vi "Stepper_test_1.vi"() -> ()   [LabVIEW 2016]
uses:
  <vilib>/myRIO/Instrument Drivers/Onboard IO/DIO/typedefs/DIO Reference.ctl
  <vilib>/myRIO/Common/Instrument Driver Framework/Utilities/typedefs/myRIO Generic Hardware Reference.ctl
  <vilib>/myRIO/Common/Instrument Driver Framework/Utilities/typedefs/Hardware Version Enum.ctl
  <vilib>/myRIO/Common/Instrument Driver Framework/Utilities/typedefs/myRIO v1.0 Reference.ctl
  <vilib>/myRIO/Common/Instrument Driver Framework/Utilities/typedefs/Generic FPGA Reference.ctl
  <vilib>/myRIO/Common/Instrument Driver Framework/myRIO v1.0/DIO/typedefs/DIO Channels List.ctl
  <vilib>/myRIO/Common/Instrument Driver Framework/myRIO v1.0/DIO/typedefs/DIO Channels Enum.ctl
  <vilib>/userdefined/High Color/nirio_resource_hc.ctl
  <vilib>/myRIO/Instrument Drivers/Onboard IO/AI/typedefs/AI Reference.ctl
  <vilib>/myRIO/Common/Instrument Driver Framework/myRIO v1.0/AI/typedefs/AI Channels List.ctl
  <vilib>/myRIO/Common/Instrument Driver Framework/myRIO v1.0/AI/typedefs/AI Channels Enum.ctl
  <vilib>/myRIO/Common/Instrument Driver Framework/Utilities/typedefs/Analog Scaling Constants List.ctl
  <vilib>/myRIO/Common/Instrument Driver Framework/Utilities/typedefs/Analog Scaling Constants.ctl
  <vilib>/myRIO/Common/Instrument Driver Framework/Utilities/vis/Is FPGA Ref Available.vi
  <vilib>/myRIO/Common/Instrument Driver Framework/myRIO v1.0/AI/vis/myRIO v1.1 Open AI.vi
  <vilib>/myRIO/Instrument Drivers/Onboard IO/AI/vis/Read.vi
  <vilib>/myRIO/Common/Instrument Driver Framework/myRIO v1.0/DIO/vis/myRIO v1.1 Open DIO.vi
  <vilib>/myRIO/Instrument Drivers/Onboard IO/DIO/vis/Write.vi
  <vilib>/myRIO/Common/Instrument Driver Framework/Utilities/vis/Validate Channels.vi
  <vilib>/myRIO/Common/Instrument Driver Framework/myRIO v1.0/AI/vis/myRIO v1.0 Reserve AI.vi
  <vilib>/myRIO/Common/Instrument Driver Framework/myRIO v1.0/DIO/vis/myRIO v1.0 Reserve DIO.vi
  <vilib>/myRIO/Common/Instrument Driver Framework/myRIO v1.0/PWM/vis/myRIO v1.1 Open PWM.vi
  <vilib>/myRIO/Common/Instrument Driver Framework/myRIO v1.0/AI/vis/myRIO v1.0 Build MUX Configuration AI.vi
  <vilib>/myRIO/Common/Instrument Driver Framework/myRIO v1.0/Resource Manager/vis/myRIO v1.0 Reserve Channel List.vi
  <vilib>/myRIO/Common/Instrument Driver Framework/myRIO v1.0/DIO/vis/myRIO v1.0 Build MUX Configuration DIO.vi
  <vilib>/myRIO/Common/Instrument Driver Framework/myRIO v1.0/PWM/vis/myRIO v1.0 Reserve PWM.vi
  <vilib>/myRIO/Common/Instrument Driver Framework/myRIO v1.0/Resource Manager/vis/myRIO v1.0 Reserve Channel.vi
  <vilib>/myRIO/Common/Instrument Driver Framework/myRIO v1.0/Resource Manager/vis/myRIO v1.0 Unreserve Channel.vi
  <vilib>/myRIO/Common/Instrument Driver Framework/myRIO v1.0/Resource Manager/vis/myRIO v1.0 Create Configuration List.vi
  <vilib>/myRIO/Common/Instrument Driver Framework/myRIO v1.0/PWM/vis/myRIO v1.0 Build MUX Configuration PWM.vi
  <vilib>/myRIO/Common/Instrument Driver Framework/myRIO v1.0/Resource Manager/vis/myRIO v1.0 Build Mutex Name.vi
  <vilib>/Utility/VariantDataType/GetNumericInfo.vi
  <vilib>/Utility/error.llb/Error Cluster From Error Code.vi
  <vilib>/myRIO/Common/Instrument Driver Framework/myRIO v1.0/myRIO v1.1 Open.vi
  <vilib>/myRIO/Common/Instrument Driver Framework/Utilities/vis/IO Manager.vi
  <vilib>/myRIO/Common/Instrument Driver Framework/Utilities/vis/Configuration Manager.vi
  <vilib>/myRIO/Common/Instrument Driver Framework/myRIO v1.0/Resource Manager/vis/myRIO v1.0 Configure IO.vi
  <vilib>/myRIO/Common/Instrument Driver Framework/myRIO v1.0/myRIO v1.0 Close.vi
  <vilib>/myRIO/Common/Instrument Driver Framework/myRIO v1.0/DIO/vis/myRIO v1.0 Write DIO.vi
  <vilib>/myRIO/Common/Instrument Driver Framework/myRIO v1.0/PWM/vis/myRIO v1.0 Write PWM.vi
  <vilib>/myRIO/Common/Instrument Driver Framework/myRIO v1.0/AI/vis/myRIO v1.0 Get Scaling Constants AI.vi
  <vilib>/myRIO/Common/Instrument Driver Framework/myRIO v1.0/AI/vis/myRIO v1.0 Read AI.vi
  <vilib>/myRIO/Express VI/Onboard IO/DO/DO Express VI.xnode
  <vilib>/myRIO/Instrument Drivers/Onboard IO/DIO/vis/myRIO DIO Open.xnode
  <vilib>/myRIO/Express VI/Onboard IO/AI/AI Express VI.xnode
  <vilib>/myRIO/Instrument Drivers/Onboard IO/AI/vis/myRIO AI Open.xnode
  <vilib>/myRIO/Instrument Drivers/Onboard IO/AI/AI.lvlib
  <vilib>/myRIO/Instrument Drivers/Onboard IO/DIO/DIO.lvlib
  <vilib>/myRIO/Instrument Drivers/Onboard IO/PWM/PWM.lvlib
panel:
  in  "Servo":bool
  in  "PWM channel":tag="B/PWM0"
  out "position [%FS]":dbl(slide) scale=0.0..180.0 scale format="%#_5g"
  out "pulse width [ms]":dbl=1.5
  out "duty cycle [%]":dbl
  out "FSR VALUE":dbl
  in  "RUN":bool
  in  "CLOSE":bool
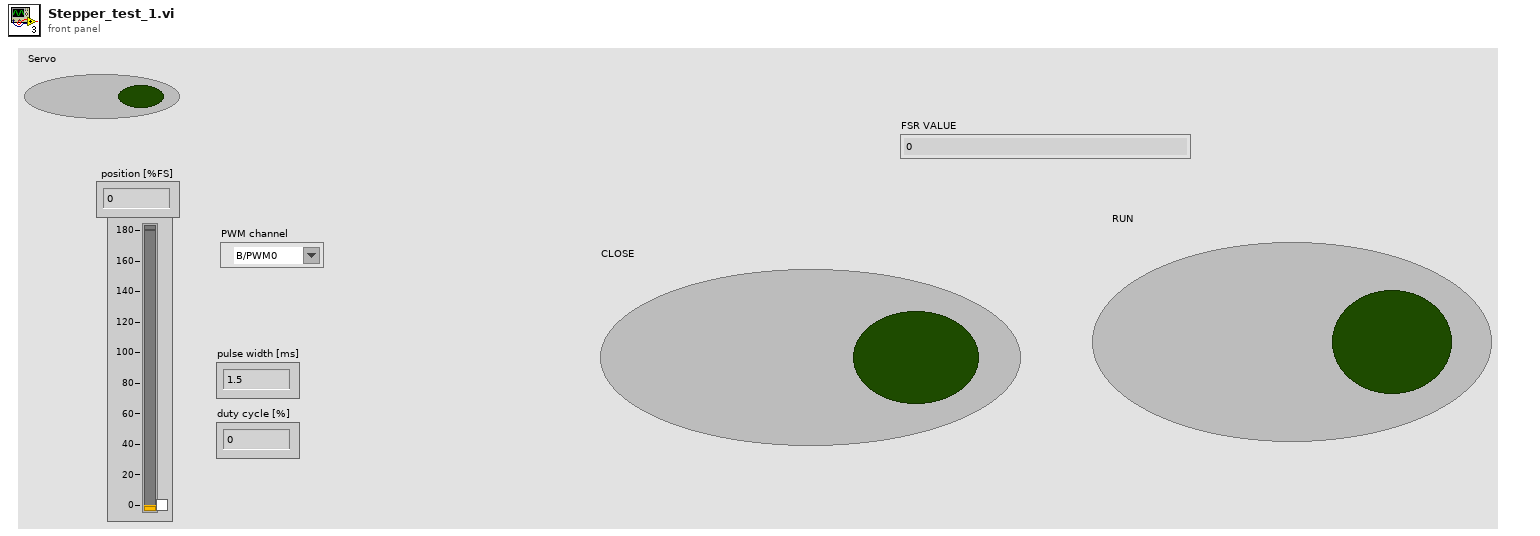
[diagram p1: front panel]
types:
  T1 = typedef "DIO.lvlib/DIO Reference.ctl" = cluster{"myRIO Reference":T2, "DIO Channels List":T6}
  T2 = typedef "myRIO Generic Hardware Reference.ctl" = cluster{"myRIO Model":T3, "myRIO Hardware Reference":T4}
  T3 = typedef "Hardware Version Enum.ctl" = enum16{"Unknown", "myRIO-1900", "myRIO-1950", "roboRIO", "NI ELVIS RIO CM"}
  T4 = typedef "myRIO v1.0 Reference.ctl" = cluster{"Generic FPGA Reference":T5, "Allow multiple opens":bool}
  T5 = typedef "Generic FPGA Reference.ctl" = refnum<k20>
  T6 = typedef "DIO Channels List.ctl" = T7[]
  T7 = typedef "DIO Channels Enum.ctl" = enum16{"Not Connected", "C/DIO0", "C/DIO1", "C/DIO2", "C/DIO3", "C/DIO4", "C/DIO5", "C/DIO6", "C/DIO7", "A/DIO0", "A/DIO1", "A/DIO2", "A/DIO3", "A/DIO4", "A/DIO5", "A/DIO6", "A/DIO7", "A/DIO8", "A/DIO9", "A/DIO10", "A/DIO11", "A/DIO12", "A/DIO13", "A/DIO14", "A/DIO15", "B/DIO0", "B/DIO1", "B/DIO2", "B/DIO3", "B/DIO4", "B/DIO5", "B/DIO6", "B/DIO7", "B/DIO8", "B/DIO9", "B/DIO10", "B/DIO11", "B/DIO12", "B/DIO13", "B/DIO14", "B/DIO15", "LED0", "LED1", "LED2", "LED3", "Button0", "DIO/DIO0", "DIO/DIO1", "DIO/DIO2", "DIO/DIO3", "DIO/DIO4", "DIO/DIO5", "DIO/DIO6", "DIO/DIO7", "DIO/DIO8", "DIO/DIO9", "SPI/CS0", "SPI/CS1", "SPI/CS2", "SPI/CS3", "LED RADIO (Green)", "LED RADIO (Red)", "LED COMM (Green)", "LED COMM (Red)", "LED MODE (Green)", "LED MODE (Red)"}
  T8 = typedef "nirio_resource_hc.ctl" = tag
  T9 = typedef "AI.lvlib/AI Reference.ctl" = cluster{"myRIO Reference":T2, "AI Channels List":T10, "AI Scaling Constants List":T12}
  T10 = typedef "AI Channels List.ctl" = T11[]
  T11 = typedef "AI Channels Enum.ctl" = enum16{"Not Connected", "AudioIn/Left", "AudioIn/Right", "C/AI0", "C/AI1", "A/AI0", "A/AI1", "A/AI2", "A/AI3", "B/AI0", "B/AI1", "B/AI2", "B/AI3", "AI/AI0", "AI/AI1", "AI/AI2", "AI/AI3"}
  T12 = typedef "Analog Scaling Constants List.ctl" = T13[]
  T13 = typedef "Analog Scaling Constants.ctl" = cluster{"LSB Weight (Volts)":dbl, "Offset (Volts)":dbl, "Signed?":bool}
  T14 = typedef "PWM.lvlib/PWM Reference.ctl" = cluster{"myRIO Reference":T2, "PWM Channels Enum":T15, "PWM Configuration":T16}
  T15 = typedef "PWM Channels Enum.ctl" = enum16{"Not Connected", "C/PWM0", "C/PWM1", "A/PWM0", "A/PWM1", "A/PWM2", "B/PWM0", "B/PWM1", "B/PWM2", "PWM/PWM0", "PWM/PWM1", "PWM/PWM2", "PWM/PWM3", "PWM/PWM4", "PWM/PWM5", "PWM/PWM6", "PWM/PWM7", "PWM/PWM8", "PWM/PWM9"}
  T16 = typedef "PWM.lvlib/PWM Configuration.ctl" = cluster{"Frequency":dbl, "Duty Cycle":dbl}
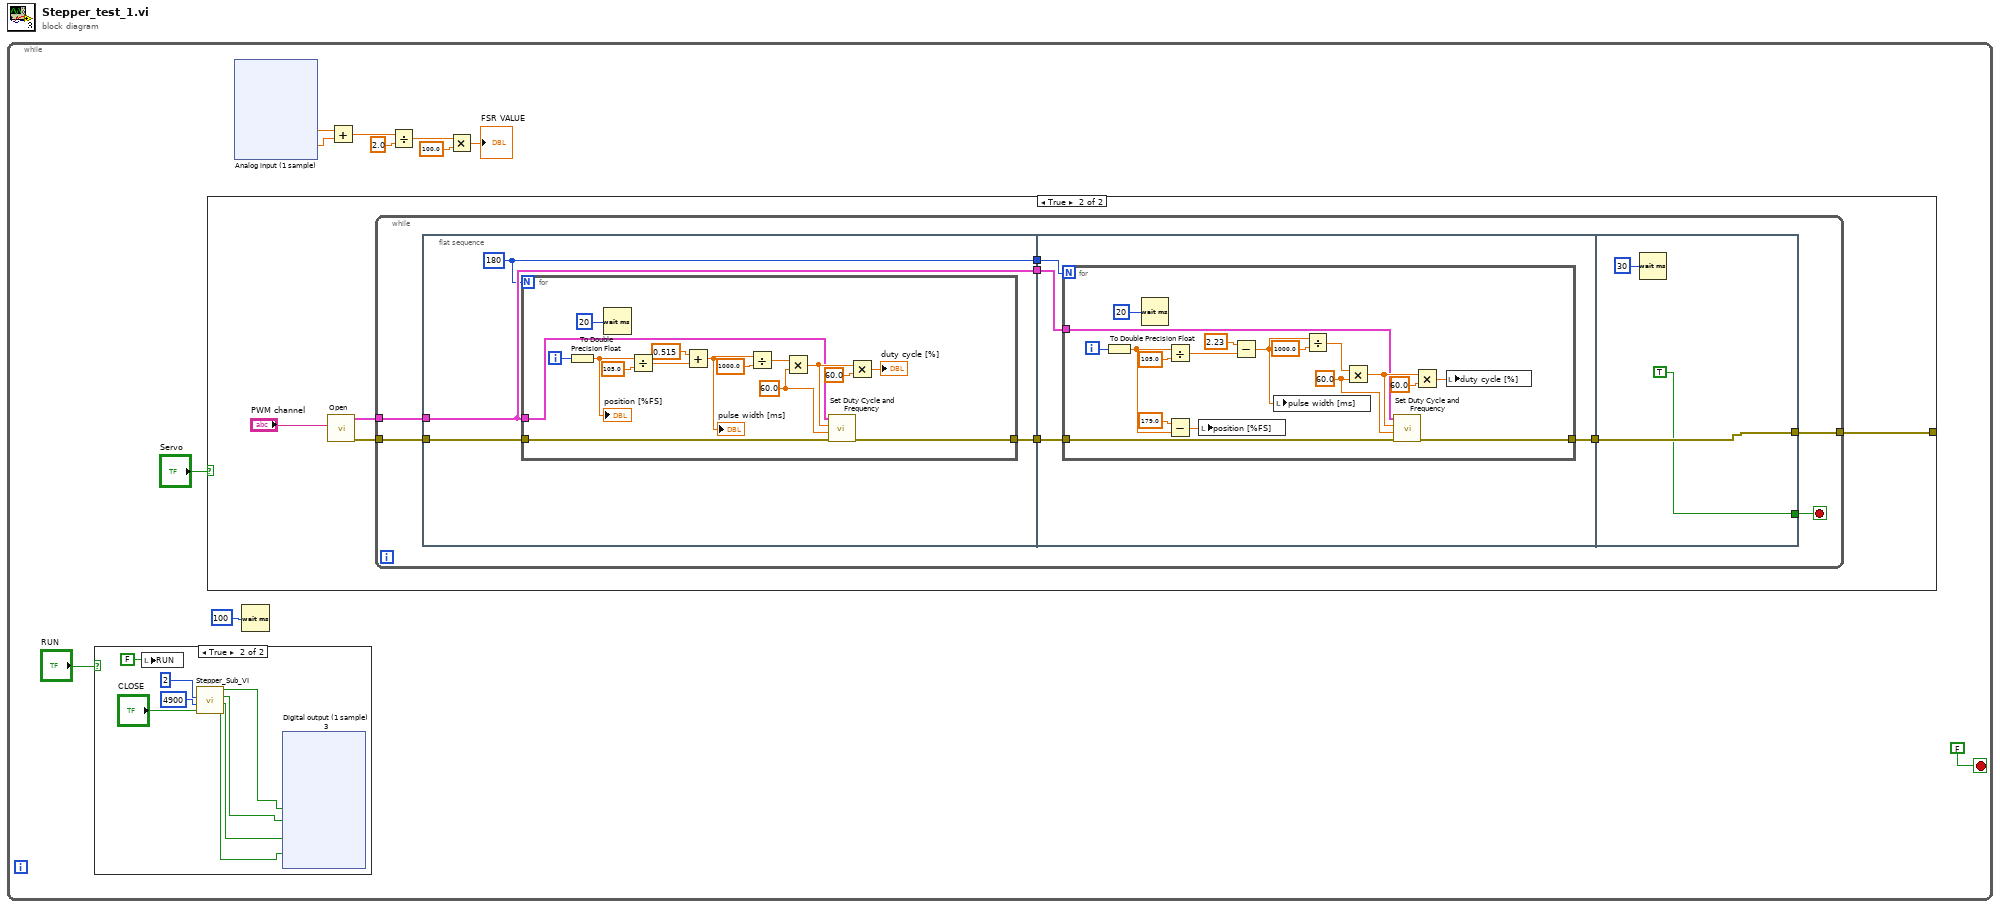
[diagram p0: block diagram]
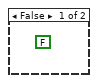
[diagram p2: hidden frame]
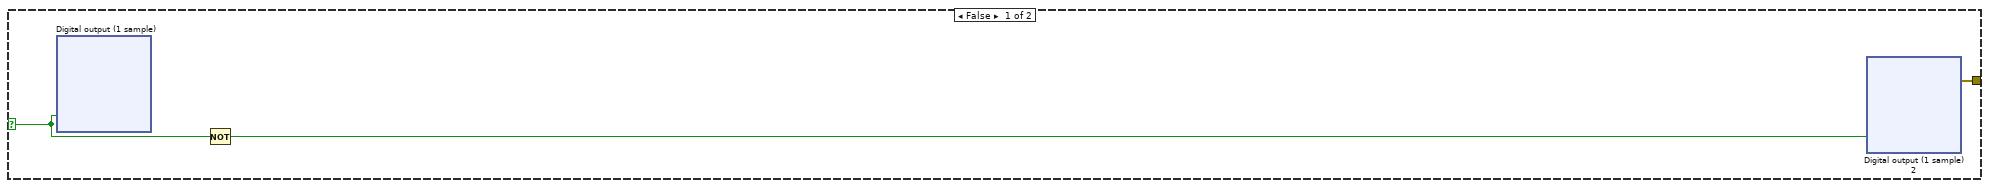
[diagram p3: hidden frame]
diagram:
  n1 = while {
    stop <- FALSE stop-if-true
    n2 = case shown="True" "RUN" {
      frame False {
        (unwired) FALSE ("Boolean")
      }
      frame True {
        n3 = local write "RUN"(FALSE ("Run")) -> ()
        n4 = call "Stepper_Sub_VI.vi"("dir"="CLOSE", "Numeric 2"=4900, "milliseconds to wait"=u32 2) -> ("FSR  RED LED"=w12:bool, "FSR   RED LED"=w13:bool, "FRS GREEN LED"=w14:bool, "FRS  GREEN LED"=w15:bool)  [unwired: 5 in]
        n5 = xnode "Digital output (1 sample) 3"("GREEN (A/DIO0 (Pin 11))"=w15, "GREEN (A/DIO1 (Pin 13))"=w14, "A/DIO5 (Pin 21)"=w13, "A/DIO6 (Pin 23)"=w12) -> ()  [unwired: 1 in, 1 out]
      }
    }
    n6 = case shown="True" "Servo" {
      selector: "Servo" -> [w58 _]
      tunnel: [w59 w132] -> _
      frame False {
        n7 = xnode "Digital output (1 sample)"("B/DIO15 (Pin 34)"=w58) -> ()  [unwired: 1 in, 1 out]
        n8 = Not(x=w58) -> (.not. x?=w60:bool)
        n9 = xnode "Digital output (1 sample) 2"("B/DIO14 (Pin 32)"=w60) -> ("error out"=w59:errorcluster)  [unwired: 1 in]
      }
      frame True {
        n10 = call <vilib>:"Open.vi"("Channel Name"="PWM channel") -> ("error out"=w131:errorcluster, "PWM Ref Out"=w133:T14)  [unwired: 9 in]
        n11 = while {
          tunnel: w133 -> [w142]
          tunnel: [w137] -> w132
          tunnel: w131 -> [w141]
          stop <- w135 stop-if-true
          n12 = flat-sequence {
            tunnel: w142 -> [w144]
            tunnel: w141 -> [w145]
            tunnel: [w146] -> w140
            tunnel: [w144] -> w139
            tunnel: [w143] -> w138
            tunnel: w140 -> [w164]
            tunnel: w139 -> [w166]
            tunnel: w138 -> [w165]
            tunnel: [w163] -> w136
            tunnel: [w186] -> w137
            tunnel: w136 -> [w186]
            tunnel: [TRUE] -> w135
            frame #0 {
              w143 = 180
              n13 = for {
                N: w143 -> [_]
                tunnel: [w158] -> w146
                tunnel: w144 -> [w150]
                tunnel: w145 -> [w147]
                i -> [w148]
                w159 = 60.0 ("freq [Hz]")
                n14 = To Double Precision Float(number=w148) -> (double precision float=w151:dbl)
                "position [%FS]" <- w151
                n15 = Wait (ms)(milliseconds to wait=u32 20) -> ()  [unwired: 1 out]
                n16 = Divide(x=w151, y=105.0) -> (x/y=w153:dbl)
                n17 = Add(x=0.515 ("y"), y=w153) -> (x+y=w149:dbl)
                "pulse width [ms]" <- w149
                n18 = Divide(x=w149, y=1000.0) -> (x/y=w157:dbl)
                n19 = Multiply(x=w157, y=w159) -> (x*y=w154:dbl)
                n20 = call <vilib>:"Set Duty Cycle and Frequency.vi"("error in (no error)"=w147, "Frequency [Hz]"=w159, "Duty Cycle"=w154, "PWM Ref In"=w150) -> ("error out"=w158:errorcluster)  [unwired: 5 in, 1 out]
                n21 = Multiply(x=w154, y=60.0) -> (x*y=→"duty cycle [%]":dbl)
              }
            }
            frame #1 {
              n22 = for {
                N: w165 -> [_]
                tunnel: [w180] -> w163
                tunnel: w164 -> [w173]
                tunnel: w166 -> [w172]
                i -> [w174]
                w181 = 60.0 ("freq [Hz]")
                n23 = To Double Precision Float(number=w174) -> (double precision float=w168:dbl)
                n24 = Wait (ms)(milliseconds to wait=u32 20) -> ()  [unwired: 1 out]
                n25 = Divide(x=w168, y=105.0) -> (x/y=w176:dbl)
                n26 = Subtract(x=179.0, y=w168) -> (x-y=w169:dbl)
                n27 = local write "position [%FS]"(w169) -> ()
                n28 = Subtract(x=2.23 ("y"), y=w176) -> (x-y=w171:dbl)
                n29 = local write "pulse width [ms]"(w171) -> ()
                n30 = Divide(x=w171, y=1000.0) -> (x/y=w179:dbl)
                n31 = Multiply(x=w179, y=w181) -> (x*y=w177:dbl)
                n32 = call <vilib>:"Set Duty Cycle and Frequency.vi"("error in (no error)"=w173, "Frequency [Hz]"=w181, "Duty Cycle"=w177, "PWM Ref In"=w172) -> ("error out"=w180:errorcluster)  [unwired: 5 in, 1 out]
                n33 = Multiply(x=w177, y=60.0) -> (x*y=w170:dbl)
                n34 = local write "duty cycle [%]"(w170) -> ()
              }
            }
            frame #2 {
              n35 = Wait (ms)(milliseconds to wait=u32 30) -> ()  [unwired: 1 out]
            }
          }
        }
      }
    }
    n36 = xnode "Analog input (1 sample)"() -> ("right fsr (A/AI0 (Pin 3))"=w10:dbl, "left fsr (A/AI1 (Pin 5))"=w9:dbl)  [unwired: 1 in, 1 out]
    n37 = Wait (ms)(milliseconds to wait=u32 100) -> ()  [unwired: 1 out]
    n38 = Add(x=w10, y=w9) -> (x+y=w8:dbl)
    n39 = Divide(x=w8, y=2.0) -> (x/y=w6:dbl)
    n40 = Multiply(x=w6, y=100.0) -> (x*y=→"FSR VALUE":dbl)
  }
